vi "SMBus Block Read.vi"(0 "DevType":i32, 1 "CommandCode":u8, 5 "DevIndex":i32, 7 "SMBUSIndex":i32, 9 "SlaveAddr":u8, 11 "error in (no error)":errorcluster, 12 "PEC":u8) -> (4 "pData":string, 6 "pByteCount":string, 8 "function return":i32, 15 "error out":errorcluster)   [LabVIEW 2012, in "ControlSMBus.lvlib"]
doc: "int WINAPI SMBus_BlockRead(int DevType,int DevIndex,int SMBUSIndex,unsigned char SlaveAddr,unsigned char CommandCode,unsigned char *pData,unsigned char *pByteCount,unsigned char PEC);"
uses:
  ControlSMBus.lvlib
  Ginkgo_Driver.dll
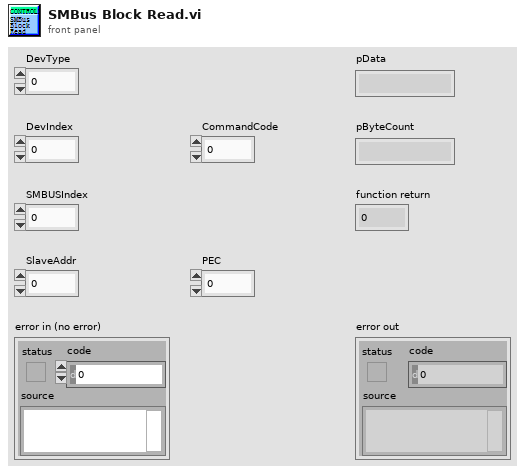
[diagram p1: front panel]
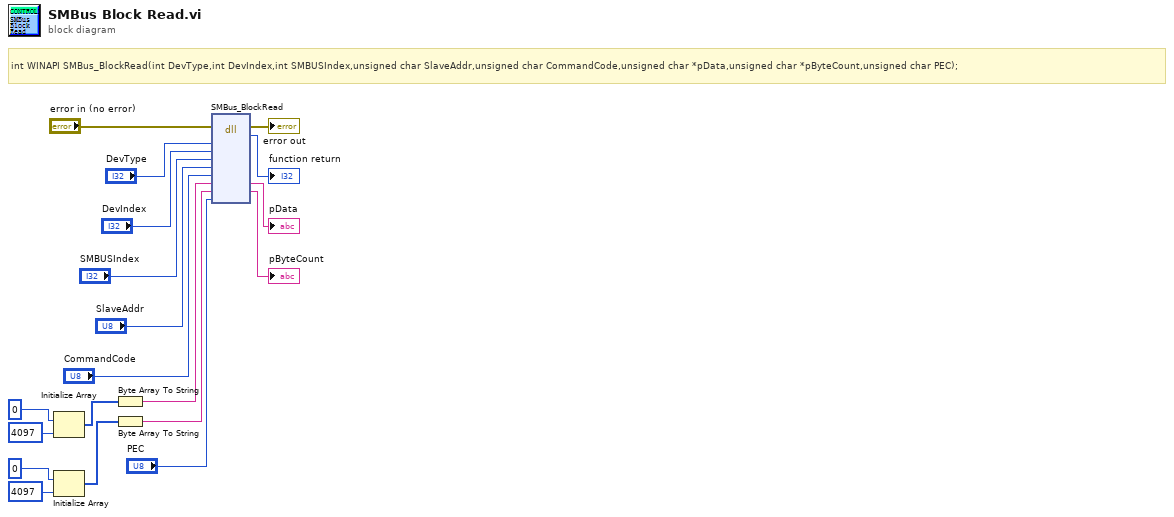
[diagram p0: block diagram]
diagram:
  # "int WINAPI SMBus_BlockRead(int DevType,int DevIndex,int SMBUSIndex,unsigned char SlaveAddr,unsigned char CommandCode,unsigned char *pData,unsigned char *pByteCount,unsigned char PEC);"
  n1 = Initialize Array(u8 0 ("element"), 4097 ("dimension size")) -> (w13:u8[])
  n2 = Initialize Array(u8 0 ("element"), 4097 ("dimension size")) -> (w8:u8[])
  n3 = Byte Array To String(unsigned byte array=w13) -> (string=w12:string)
  n4 = Byte Array To String(unsigned byte array=w8) -> (string=w7:string)
  n5 = dll-call lib="E:/Project/vt_ginkgo/truck/Ginkgo Driver/vs2010/Ginkgo_USB-I2C_API_v2.0.3.0/lib/labview_64bit/ControlSMBus/Ginkgo_Driver.*" fn="SMBus_BlockRead"(error in="error in (no error)", "DevType"="DevType", "DevIndex"="DevIndex", "SMBUSIndex"="SMBUSIndex", "SlaveAddr"="SlaveAddr", "CommandCode"="CommandCode", "pData"=w12, "pByteCount"=w7, "PEC"="PEC") -> (error out=→"error out":errorcluster, →"function return":i32, "pData"=→"pData":string, "pByteCount"=→"pByteCount":string)  [unwired: 8 in, 1 out]
